vi "Configure Digital Output Port.vi"(8 "Error In":errorcluster, 10 "DO Pins":u8[](array[numeric]), 11 "ChipKit Resource":T1={"COM Port"="", "Board Type"=enum."ChipKit uC32", "Connection Type"=enum."USB / Serial", "Baud Rate (115200)"=15, "Bytes Per Packet (15)"=15}) -> (0 "Error Out":errorcluster, 3 "ChipKit Resource":T1={"COM Port"="", "Board Type"=enum."ChipKit uC32", "Connection Type"=enum."USB / Serial", "Baud Rate (115200)"=15, "Bytes Per Packet (15)"=15})   [LabVIEW 2011, in "LabVIEW Interface for ChipKit.lvlib"]
doc: "Configure a set of digital pins as outputs. After configuring the pins with this VI use the Digital Write Port VI to write a value to each configured pin in a single operation."
uses:
  LabVIEW Interface for ChipKit.lvlib
  Private/Type Defs/Command.ctl
  Private/Type Defs/Board Type.ctl
  Private/Type Defs/Connection Type.ctl
  Private/Type Defs/Chipkit Resource.ctl
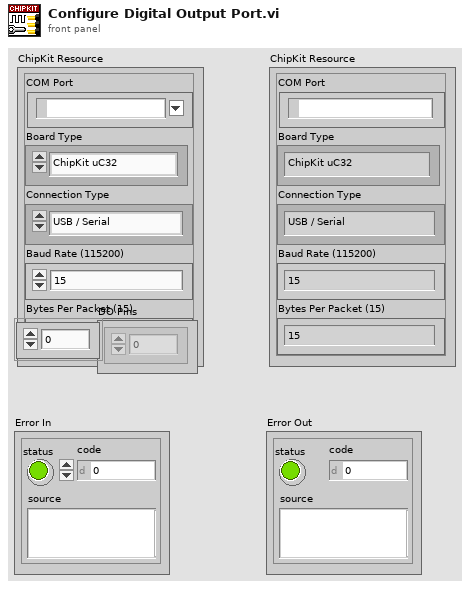
[diagram p1: front panel]
types:
  T1 = typedef "LabVIEW Interface for ChipKit.lvlib/Chipkit Resource.ctl" = cluster{"COM Port":refnum<visa-resource-name>, "Board Type":T2, "Connection Type":T3, "Baud Rate (115200)":u32, "Bytes Per Packet (15)":u32}
  T2 = typedef "LabVIEW Interface for ChipKit.lvlib/Board Type.ctl" = enum16{"ChipKit uC32", "ChipKit Uno32", "ChipKit Max32"}
  T3 = typedef "LabVIEW Interface for ChipKit.lvlib/Connection Type.ctl" = enum8{"USB / Serial", "XBEE", "BlueSmirf (Bluetooth)"}
  T4 = typedef "LabVIEW Interface for ChipKit.lvlib/Command.ctl" = enum8{"setArduinoMode", "flushSerial", "setPinMode", "digitalWritePin", "digitalWritePort", "tone", "digitalReadPin", "digitalReadPort", "analogReadPin", "analogReadPort", "pwmWritePin", "pwmWritePort", "sevenSegment_Configure", "sevenSegment_Write", "I2C Init", "I2C Write", "I2C Read", "SPI Init", "SPI Set Bit Order", "SPI Set Clock Divider", "SPI Set Data Mode", "SPI Send / Receive", "SPI Close", "Servo Set Num Servos", "Servo Config Servo", "Servo Write Angle", "Servo Read Angle", "Servo Write Pulse Width", "Servo Read Pulse Width", "Servo Detach", "LCD Init", "LCD Set Size", "LCD Set Cursor Mode", "LCD Clear", "LCD Set Cursor Position", "LCD Print", "LCD Display Power", "LCD Scroll Display", "LCD Autoscroll", "LCD Print Direction", "LCD Create Custom Char", "LCD Print Custom Char", "contAcqOn", "contAcqOff", "getFirmwareVersion", "FiniteSampleStart", "NA", "NA2", "Conifg Stepper", "Stepper Write", "Stepper Detach", "Stepper Steps To Go", "Config DO Port", "Config DI Port", "UART2 Open", "UART2 Write", "UART2 Bytes Available", "UART2 Read"}
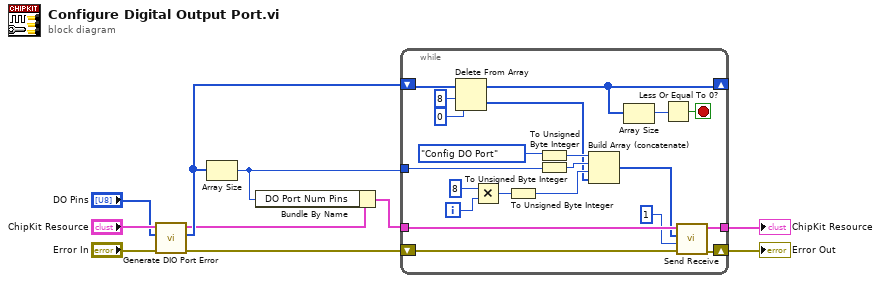
[diagram p0: block diagram]
diagram:
  n1 = call "Generate DIO Port Error.vi"("Error in"="Error In", "DO Pins"="DO Pins", "ChipKit Resource"="ChipKit Resource") -> ("Error Out"=w7:errorcluster, "DO Pins"=w4:u8[], "ChipKit Resource"=w2:T1)  [unwired: 6 in]
  n2 = Array Size(array=w4) -> (size(s)=w3:i32)
  n3 = Bundle By Name(cluster=w2, "DO Port Num Pins"=w3) -> (w1:T1)
  n4 = while {
    tunnel: w1 -> [w31]
    tunnel: [w29] -> w10
    shift-right: [w27] -> w9
    shift-left: w7 -> [w30]
    shift-right: [w14] -> _
    shift-left: w4 -> [w26]
    tunnel: w3 -> [w19]
    i -> [w17]
    stop <- w12 stop-if-true
    n5 = Delete From Array(array=w26, length=8, index=0) -> (deleted portion=w11:u8[], array with subset deleted=w14:u8[])
    n6 = Multiply(x=8, y=w17) -> (x*y=w18:i32)
    n7 = To Unsigned Byte Integer(number=w18) -> (unsigned 8bit integer=w15:u8)
    n8 = To Unsigned Byte Integer(number=Command."Config DO Port" ("Command")) -> (unsigned 8bit integer=w23:u8)
    n9 = To Unsigned Byte Integer(number=w19) -> (unsigned 8bit integer=w20:u8)
    n10 = Build Array (concatenate)(w23, w20, w15, w11) -> (w21:u8[])
    n11 = Array Size(array=w14) -> (size(s)=w13:i32)
    n12 = Less Or Equal To 0?(x=w13) -> (x <= 0?=w12:bool)
    n13 = call "Send Receive.vi"("Error In"=w30, "Bytes To Read (0)"=u8 1, "Data"=w21, "ChipKit Resource"=w31) -> ("Error Out"=w27:errorcluster, "ChipKit Resource"=w29:T1)  [unwired: 5 in, 1 out]
  }
  "Error Out" <- w9
  "ChipKit Resource" <- w10
